vi "Build Export Array.vi"(9 "Absorbance Array":dbl[](array[numeric]), 10 "Voltage Array":dbl[](array[numeric]), 11 "Time Array":dbl[](array[numeric])) -> (3 "Data Out":dbl[][](array[numeric]))   [LabVIEW 2016]
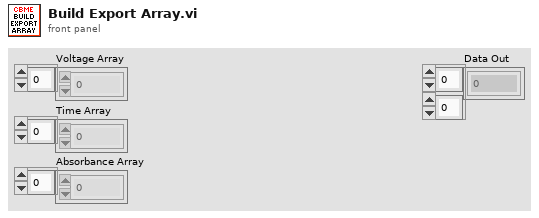
[diagram p1: front panel]
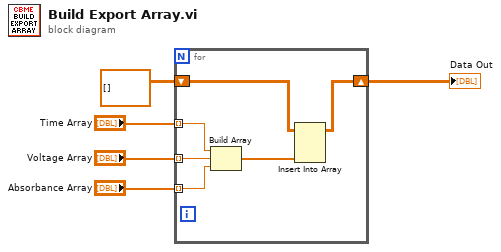
[diagram p0: block diagram]
diagram:
  n1 = for {
    tunnel: "Time Array" -> [w10] mode=indexing
    tunnel: "Voltage Array" -> [w11] mode=indexing
    tunnel: "Absorbance Array" -> [w9] mode=indexing
    shift-right: [w6] -> w1
    shift-left: dbl[][] [] ("Data") -> [w7]
    n2 = Build Array(w10, w11, w9) -> (w8:dbl[])
    n3 = Insert Into Array(array=w7, new element=w8) -> (w6:dbl[][])  [unwired: 2 in]
  }
  "Data Out" <- w1
